vi "Read T.vi"(11 "PID SP Limiter in":refnum<class "PID SP Limiter.lvclass">) -> (2 "T":u32, 3 "PID SP Limiter out":refnum<class "PID SP Limiter.lvclass">)   [LabVIEW 2019, in "control.lvlib" / "PID SP Limiter.lvclass"]
uses:
  PID SP Limiter.lvclass
  PID SP Limiter.lvclass/PID SP Limiter.ctl
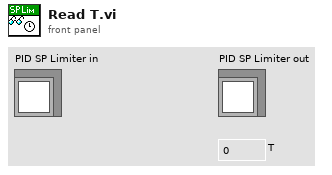
[diagram p1: front panel]
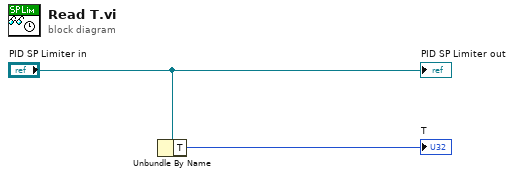
[diagram p0: block diagram]
diagram:
  n1 = Unbundle By Name("PID SP Limiter in") -> ("T"=→"T":u32)
  "PID SP Limiter out" <- "PID SP Limiter in"
